vi "FormCalibra6.vi"() -> ()   [LabVIEW 2014]
uses:
  testMachine.ctl
  mainMachine.ctl
  <vilib>/Analysis/baseanly.llb/Mean (DBL).vi
  <vilib>/express/express shared/transition.llb/Dynamic To Waveform Array.vi
  <vilib>/express/express signal manip/GetorSetDDTAttributes/Set DDT Attributes/SetT0.vi
  <vilib>/express/express shared/transition.llb/Waveform Array To Dynamic.vi
  <vilib>/measure/mamon.llb/Trigger Detection for 1 Channel.vi
  <vilib>/express/express signal manip/GetorSetDDTAttributes/Set DDT Attributes/Set DDT Properties.xnode
  <vilib>/Analysis/NI_AALBase.lvlib
  <resource>/objmgr/daqmx.rc
  <vilib>/measure/NI_MAPro.lvlib
panel:
  in  "Lower level":dbl
  in  "hysteresis":dbl format="%.2p"
  in  "level":dbl format="%.2p"
  out "rpm":bool
  out "deviceName":tag
  out "editTotalWaitLimit":u8
  out "editCountWaitLimit":u8
  out "ledWaitState":bool caption="Wait State"
  out "sliderWaitUpperTime":u8(slide) max=50 scale=0.0..100.0
  out "slideWaitLowerTime":u8(slide) max=30 scale=0.0..100.0
  out "slideWaitTime":u8(slide) scale=0.0..100.0
  out "labelTestTime":string caption="Tempo total de ensaio"
  in  "buttonAcquisition":bool
  in  "editSetWaitTime":u8 caption="Tempo entre ciclos (s)" step=1 format="%0d"
  in  "stop":bool
  out "error out":errorcluster
  out "ledAcquireState":bool caption="Acquire State"
  out "editTotalLowerLimit":u8
  out "editCountLowerLimit":u8
  out "editTotalUpperLimit":u8
  out "editCountUpperLimit":u8
  out "ledEnsaio 3":bool
  out "ledBrakeState":bool caption="Brake State"
  out "ledExitState":bool caption="Exit State"
  out "ledMotorState":bool caption="Motor State"
  out "ledInit2State":bool caption="Init State"
  out "ledBlockState":bool caption="Block State"
  out "ledRunningState":bool caption="Running State"
  out "ledReadyState":bool caption="Ready State"
  out "ledInitState":bool caption="Init State"
  out "mainMachine":T1
  out "testMachine":T2=enum."finish"
  in  "editSetPathToFile":path
  in  "buttonStop":bool
  in  "buttonStart":bool
  out "graphForce":dynamicdata(graph)
  in  "editOffsetForce":dbl caption="Tara" min=0.0 max=100.0 step=0.1
  in  "editSetForce":dbl caption="Fator de conversão"
  out "editForce":dbl caption="Força (Kgf)" format="%#_4f"
  out "graphSpeed":dynamicdata(graph)
  in  "editSetSpeed":dbl caption="Fator de conversão"
  out "editSpeed":dbl caption="Velocidade (km/h)" format="%#_4f"
  out "editEngineSpeed":dbl caption="Rotação (RPM)" format="%#_4f"
  in  "buttonMotor":bool
  in  "buttonBrake":bool
  in  "editSetWaitLowerTime":u8 caption="Tempo de espera (s)"
  in  "editSetWaitUpperTime":u8=3 caption="Tempo de espera (s)"
  in  "editSetNumberOfCycles":u16 caption="Número de ciclos" max=999 step=1 format="%0d"
  in  "editSetLowerLimit":u32 caption="Limite inferior (km/h)"
  in  "editSetUpperLimit":u32 caption="Limite superior (km/h)"
  out "editTempB":dbl caption="Temperatura B (ºC)"
  out "editTempA":dbl caption="Temperatura A (ºC)"
  in  "editSetTempRef":dbl caption="Offset referência" step=0.01 format="%#_2f"
  out "editTempRef":dbl caption="Referência (ºC)"
  out "ledMotor":bool
  out "ledBrake":bool
  out "ledEnsaio":bool
  out "labelTotalCycle":string
  out "labelCurrentCycle":string
  out "labelSystemTitle":string
  in  "editCurrCycleCtr":u32
  in  "velocidade 2":u32
  out "velocidade":u32
  # "Bancada de Frenagem - Ensaio"
  # "Ensaio"
  # "Temperatura"
  # "Rotação"
  # "Célula de Carga"
  # "Configurações do ensaio"
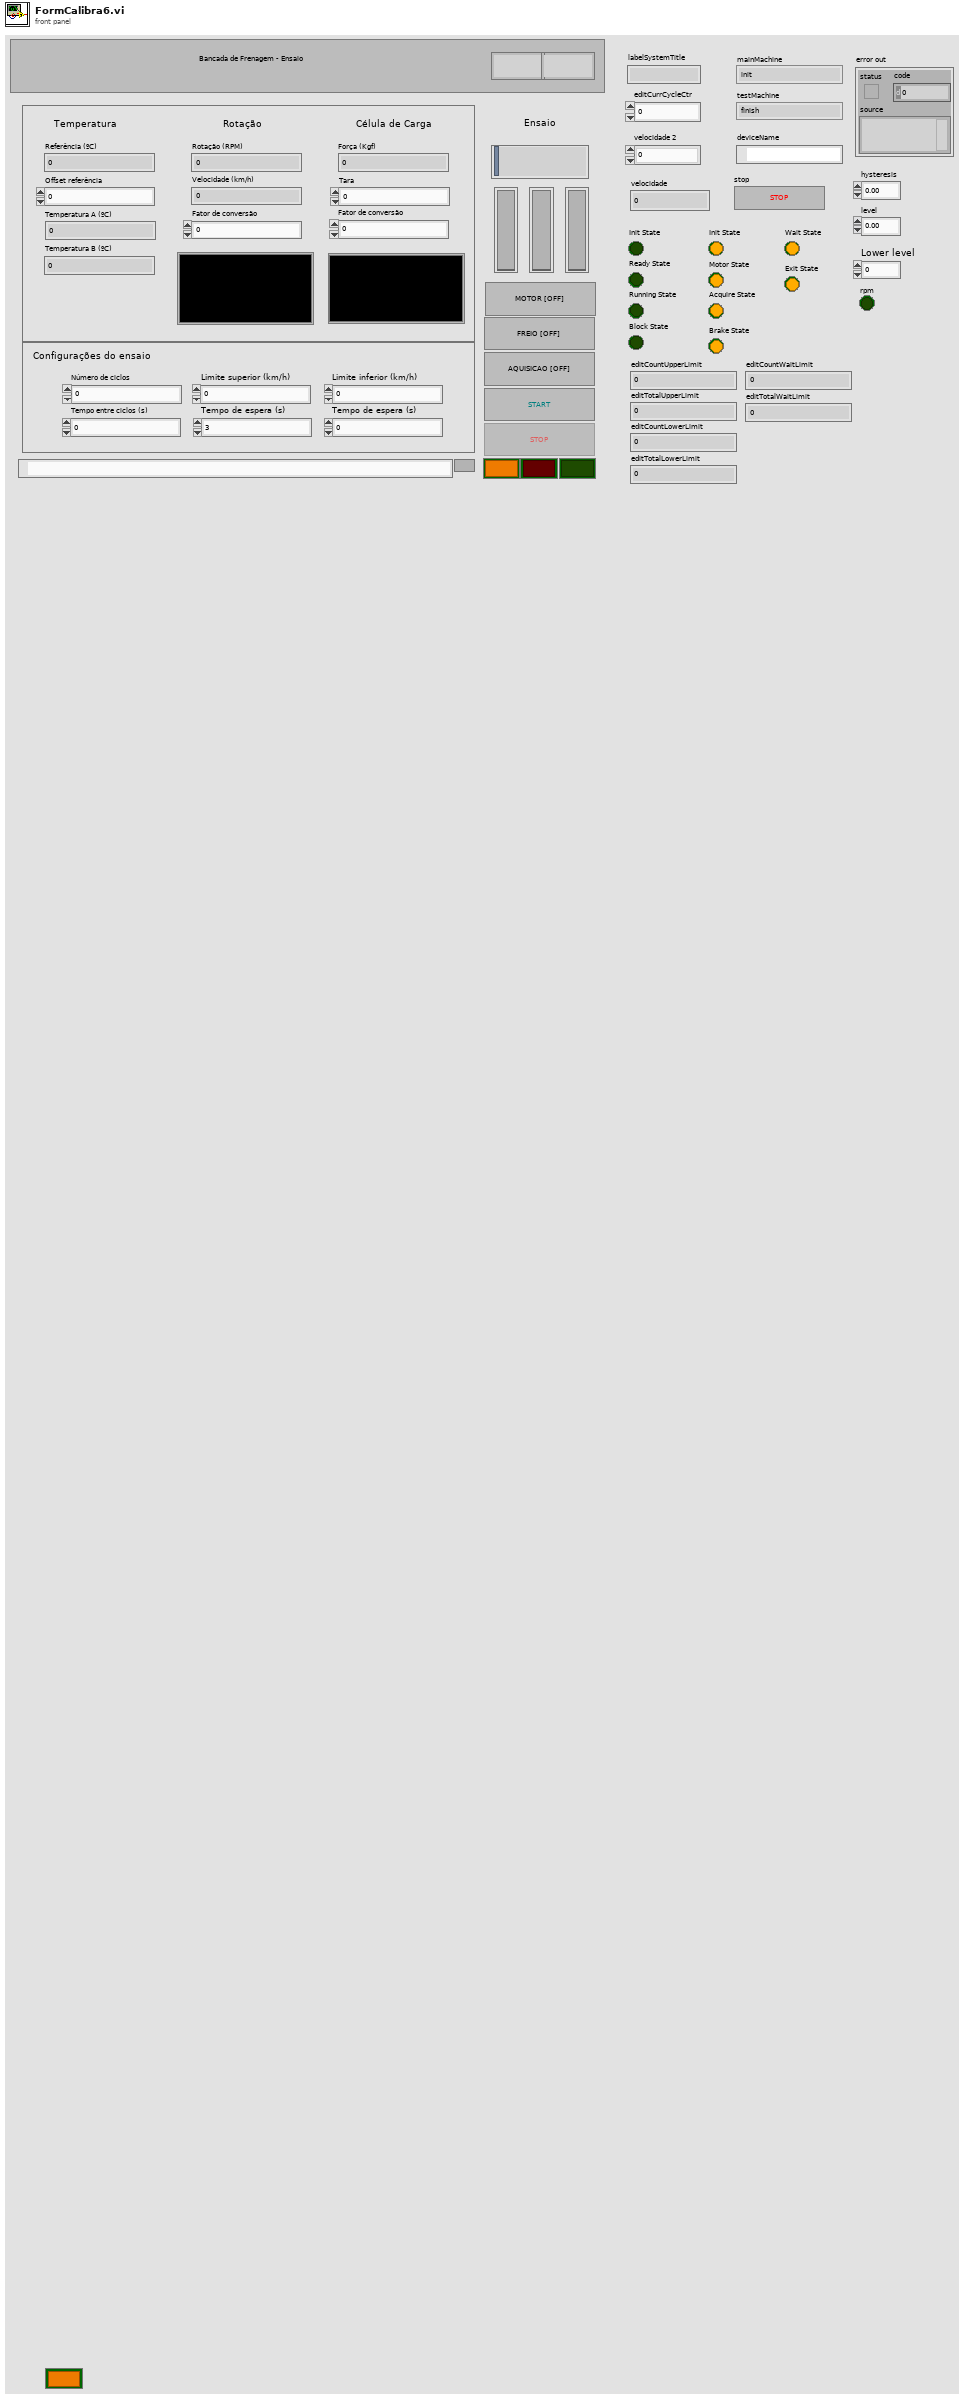
[diagram p1: front panel]
types:
  T1 = typedef "mainMachine.ctl" = enum16{"init", "ready", "running", "blocked", "finish"}
  T2 = typedef "testMachine.ctl" = enum16{"init", "motor", "motor acquire", "brake", "brake acquire", "wait ", "finish", "exit"}
  T3 = enum8{"Enabled", "Disabled", "Disabled and Grayed Out"}
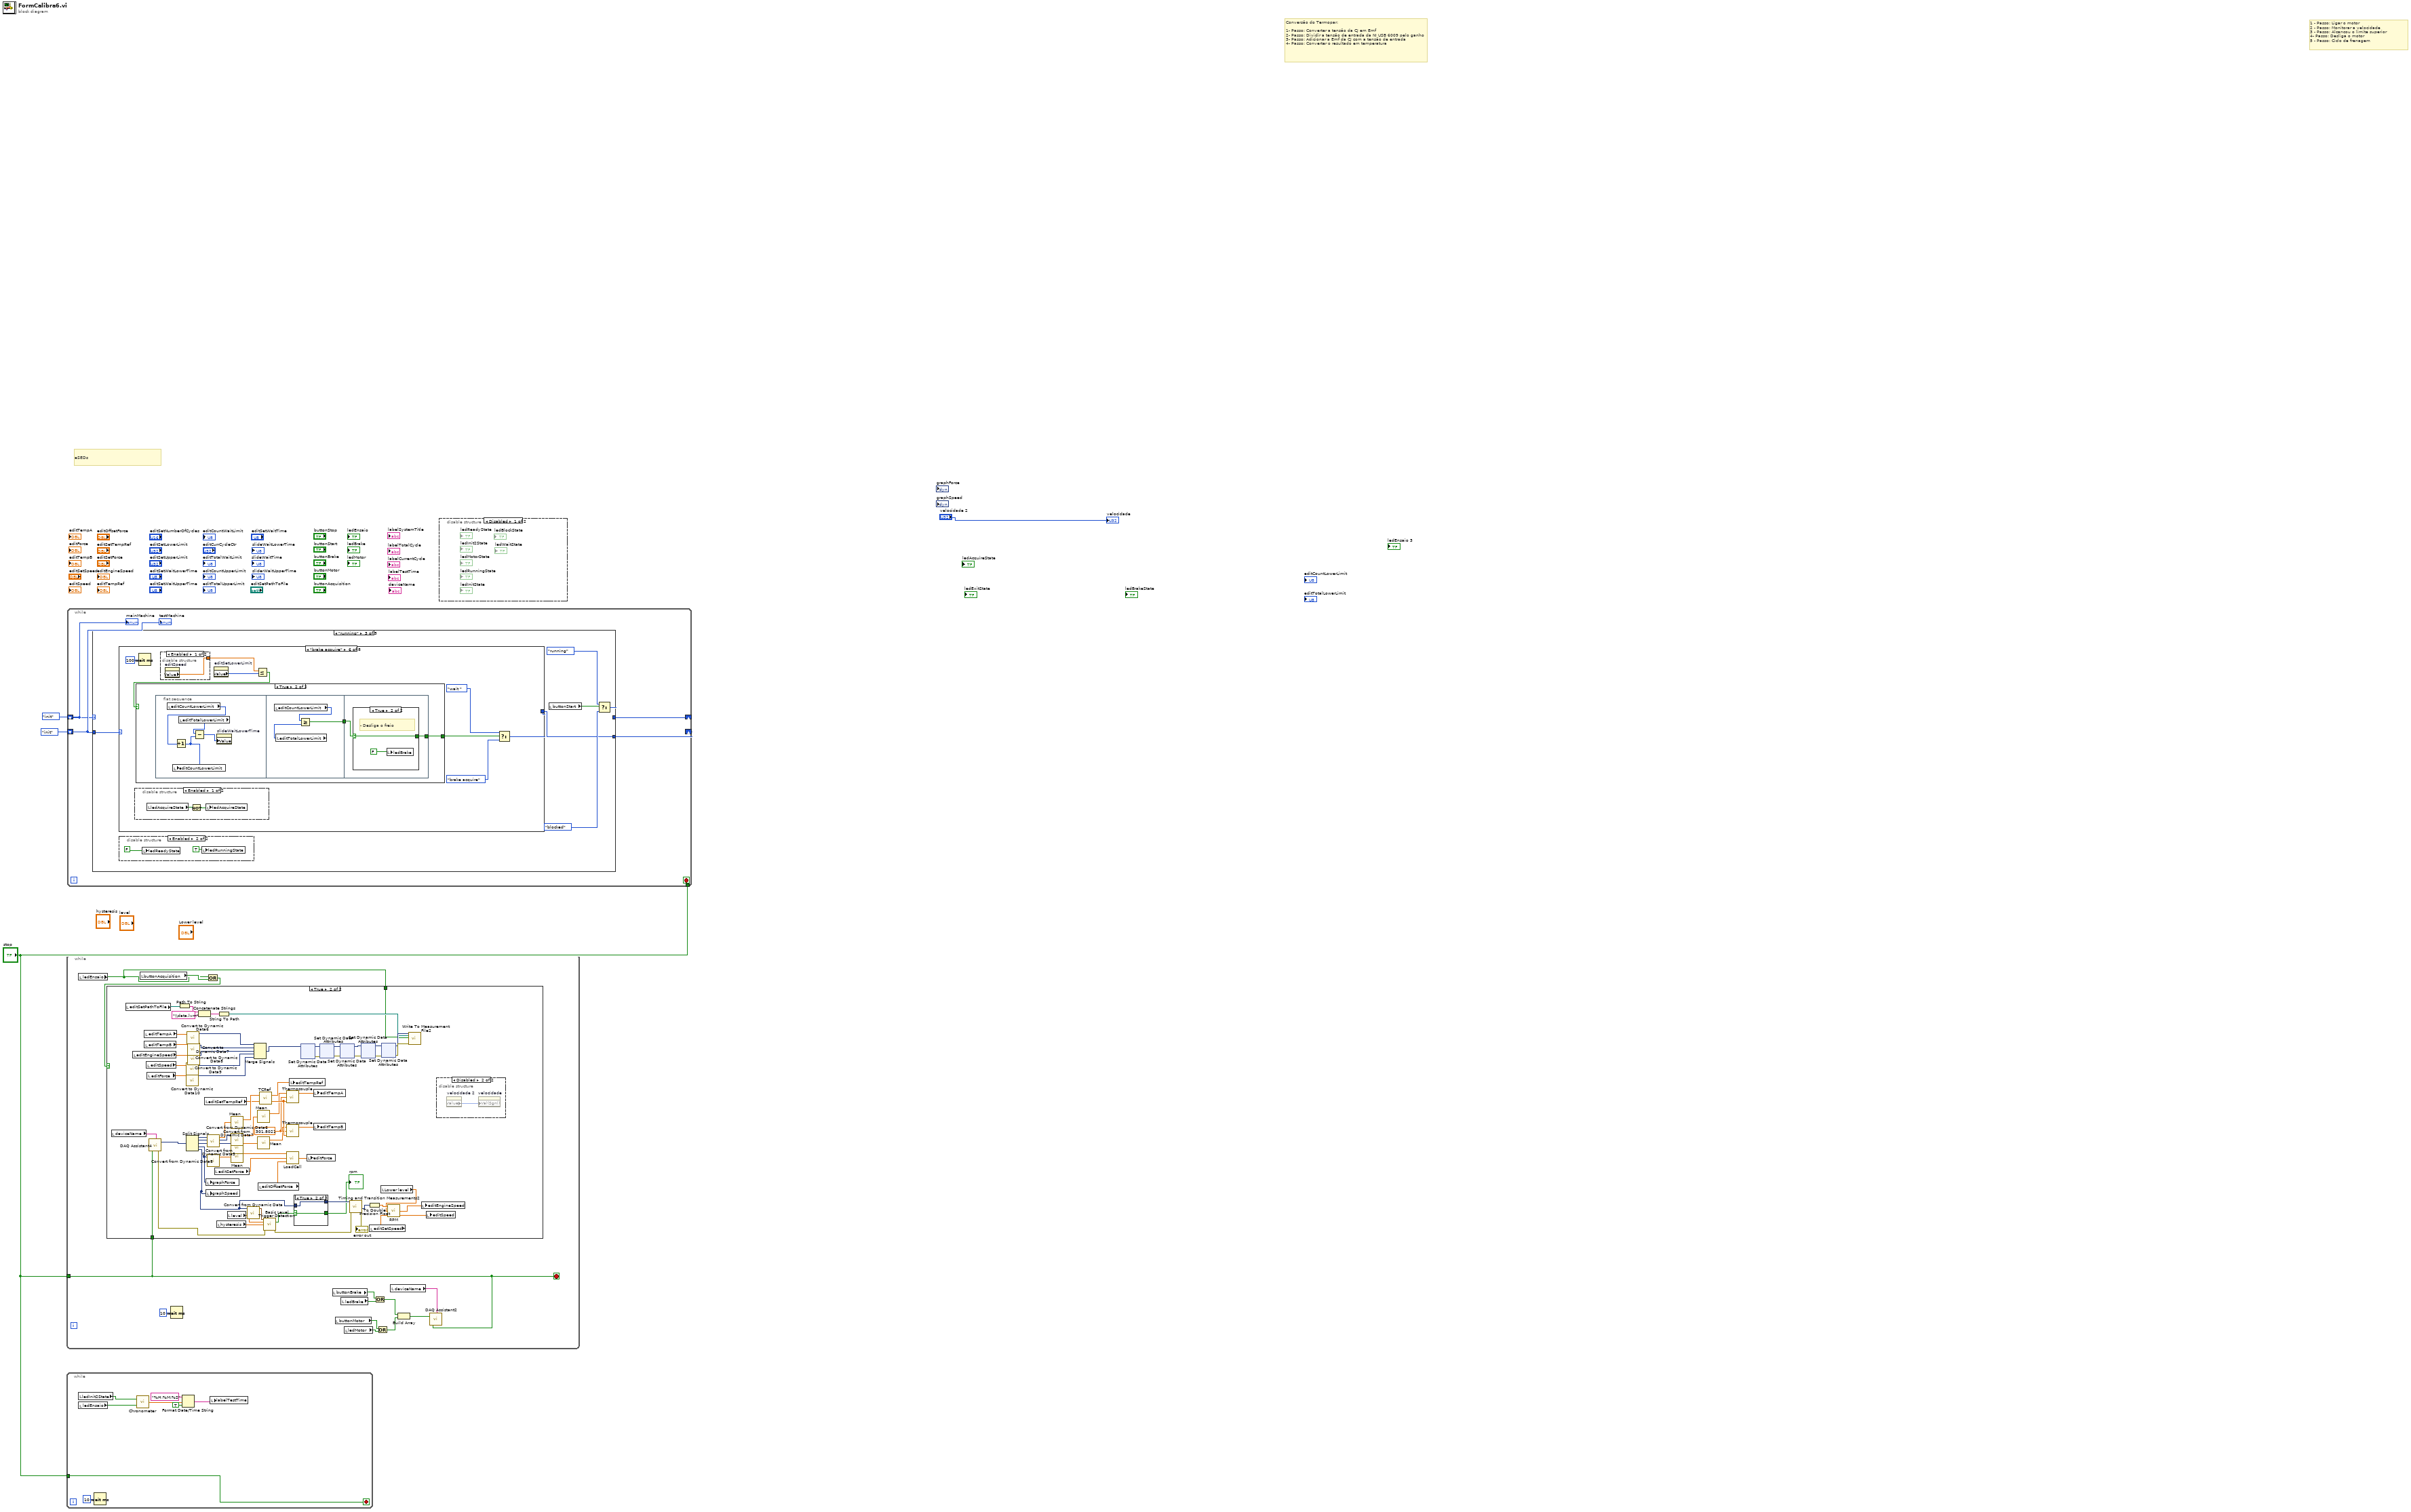
[diagram p0: block diagram]
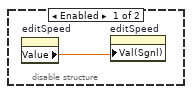
[diagram p5: hidden frame]
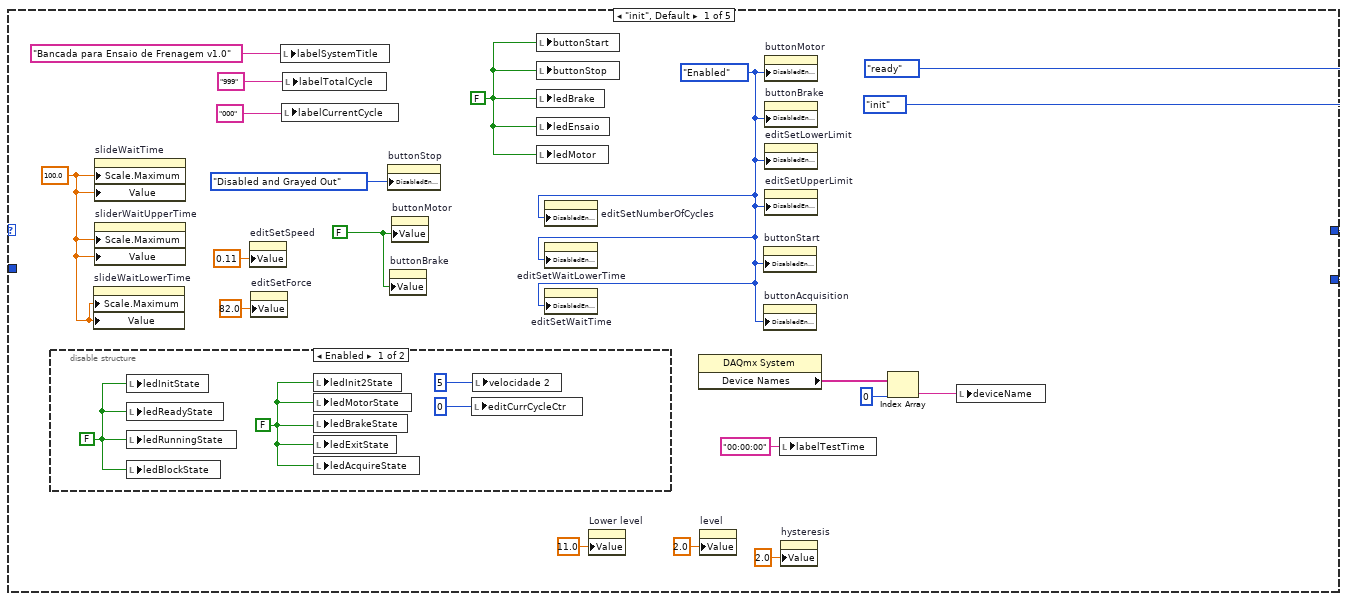
[diagram p6: hidden frame]
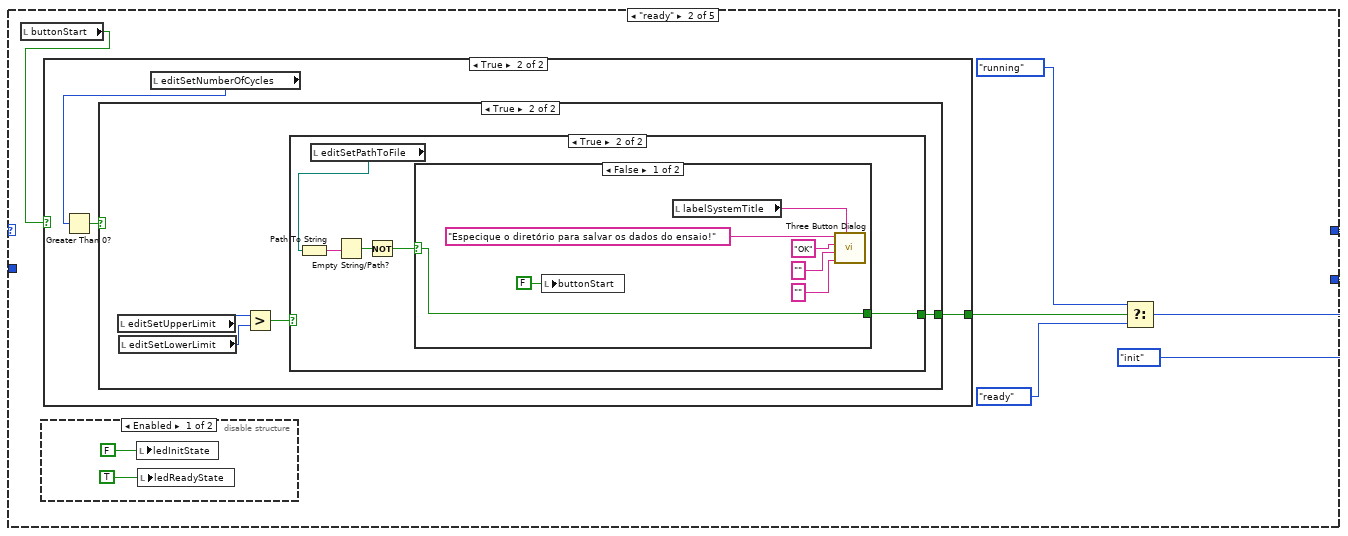
[diagram p8: hidden frame]
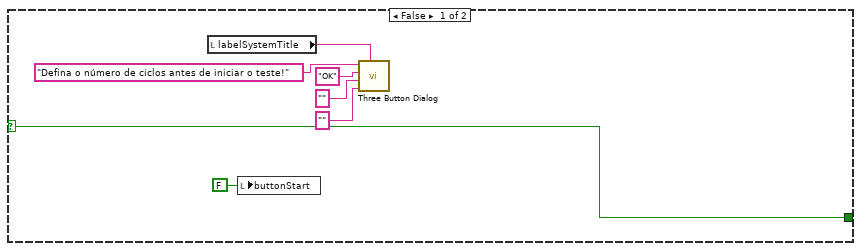
[diagram p11: hidden frame]
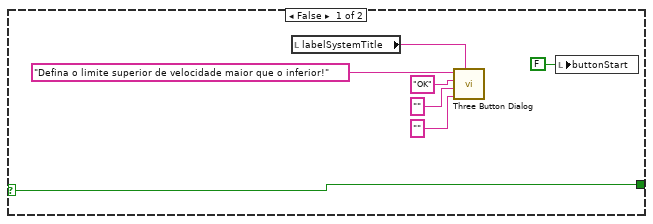
[diagram p12: hidden frame]
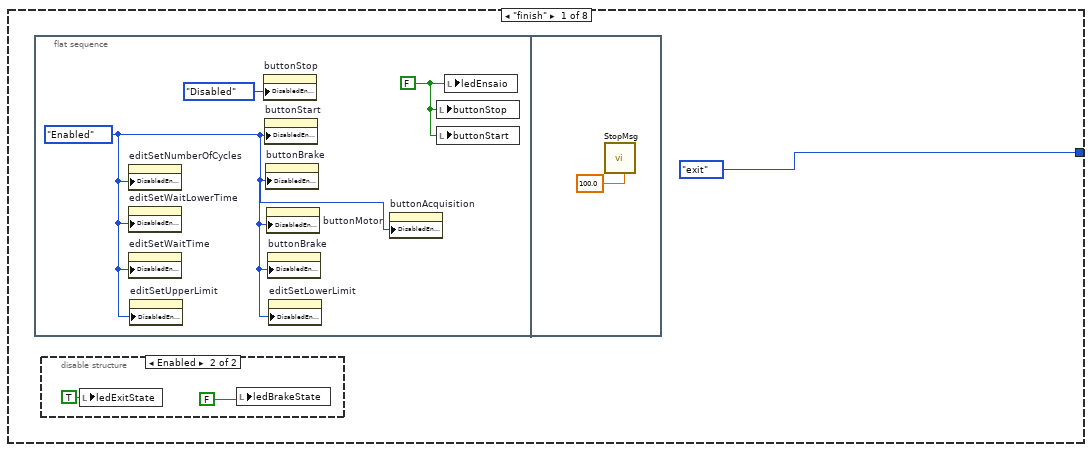
[diagram p15: hidden frame]
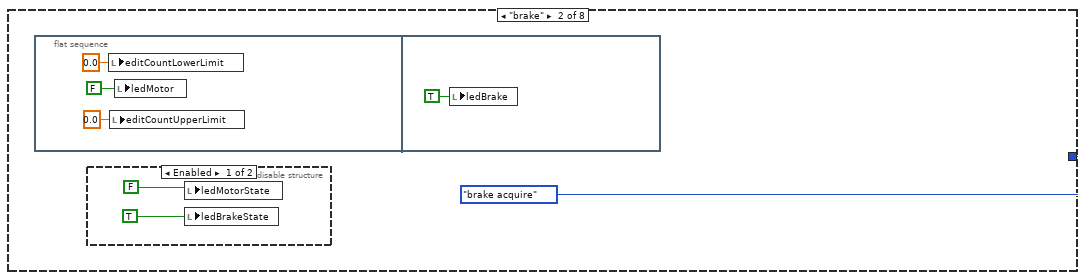
[diagram p17: hidden frame]
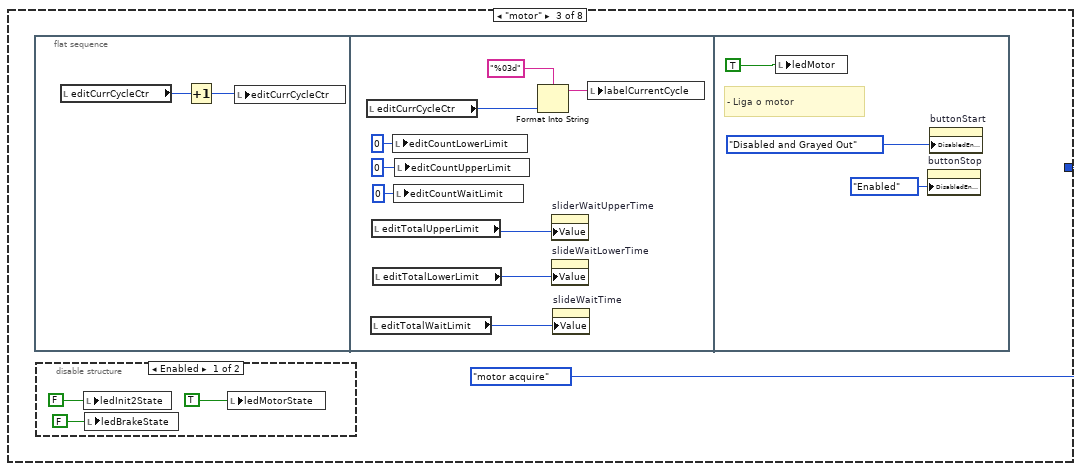
[diagram p19: hidden frame]
diagram:
  # "eSEDs"
  # "1 - Passo: Ligar o motor\n2 - Passo: Monitorar a velocidade\n3 - Passo: Alcancou o limite superior\n4- Passo: Desliga o motor\n5 - Passo: Ciclo de frenagem"
  # "Conversão do Termopar:\n\n1- Passo: Converter a tensão da CJ em Emf\n2- Passo: Dividir a tensão de entrada da NI USB 6009 pelo ganho\n3- Passo: Adicionar a Emf da CJ com a tensão de entrada\n4- Passo: Converter o resultado em temperatura"
  n1 = while {
    tunnel: "stop" -> [w12]
    stop <- w12 stop-if-true
    n2 = local read "ledInit2State"() -> (w6:bool)
    n3 = local read "ledEnsaio"() -> (w5:bool)
    n4 = Wait (ms)(milliseconds to wait=u32 10) -> ()  [unwired: 1 out]
    n5 = call "Chronometer.vi"("start"=w5, "reset"=w6) -> ("Time"=w10:dbl)
    n6 = Format Date/Time String(time format string (%c)="%H:%M:%S", seconds (now)=w10, UTC format=TRUE) -> (date/time string=w7:string)
    n7 = local write "labelTestTime"(w7) -> ()
  }
  n8 = while {
    tunnel: "stop" -> [w18]
    stop <- w18 stop-if-true
    n9 = local read "ledEnsaio"() -> (w15:bool)
    n10 = local read "buttonAcquisition"() -> (w17:bool)
    n11 = Wait (ms)(milliseconds to wait=u32 10) -> ()  [unwired: 1 out]
    n12 = Or(x=w15, y=w17) -> (x .or. y?=w16:bool)
    n13 = case shown="True" w16 {
      tunnel: w18 -> [_ w40]
      tunnel: w15 -> [_ w39]
      frame False {
      }
      frame True {
        w53 = 301.8021 ("factor")
        n14 = local read "deviceName"() -> (w38:tag)
        n15 = local read "editSetPathToFile"() -> (w68:path)
        n16 = local read "editEngineSpeed"() -> (w83:dbl)
        n17 = local read "editTempA"() -> (w80:dbl)
        n18 = local read "editTempB"() -> (w82:dbl)
        n19 = local read "editSpeed"() -> (w84:dbl)
        n20 = local read "editForce"() -> (w85:dbl)
        n21 = call "DAQ Assistant4"("stop (F)"=w40, "device name"=w38) -> ("data"=w42:dynamicdata, "error out"=w37:errorcluster)  [unwired: 14 in, 2 out]
        n22 = Path To String(path=w68) -> (string=w67:string)
        n23 = call "Convert to Dynamic Data9"("Double"=w84) -> ("Dynamic Data Type"=w88:dynamicdata)  [unwired: 3 in]
        n24 = call "Convert to Dynamic Data10"("Double"=w85) -> ("Dynamic Data Type"=w89:dynamicdata)  [unwired: 3 in]
        n25 = Split Signals(w42) -> (w45:dynamicdata, w49:dynamicdata, w47:dynamicdata, w58:dynamicdata, w34:dynamicdata)  [unwired: 5 in]
        n26 = call "Convert to Dynamic Data6"("Double"=w80) -> ("Dynamic Data Type"=w81:dynamicdata)  [unwired: 3 in]
        n27 = call "Convert to Dynamic Data7"("Double"=w82) -> ("Dynamic Data Type"=w86:dynamicdata)  [unwired: 3 in]
        n28 = call "Convert to Dynamic Data8"("Double"=w83) -> ("Dynamic Data Type"=w87:dynamicdata)  [unwired: 3 in]
        n29 = Concatenate Strings(w67, "\\data.lvm" ("string")) -> (w70:string)
        n30 = local read "editSetTempRef"() -> (w44:dbl)
        n31 = local write "graphForce"(w58) -> ()
        n32 = local write "graphSpeed"(w34) -> ()
        n33 = call "Convert from Dynamic Data5"("Dynamic Data Type"=w45) -> ("Array"=w65:dbl[])  [unwired: 3 in]
        n34 = call "Convert from Dynamic Data8"("Dynamic Data Type"=w58) -> ("Array"=w50:dbl[])  [unwired: 3 in]
        n35 = local read "editSetForce"() -> (w63:dbl)
        n36 = local read "hysteresis"() -> (w28:dbl)
        n37 = String To Path(string=w70) -> (path=w71:path)
        n38 = local read "level"() -> (w27:dbl)
        n39 = call-poly <vilib>:"Mean.vi"("X"=w65) -> ("mean"=w66:dbl)  [unwired: 1 out]
        n40 = call "Convert from Dynamic Data6"("Dynamic Data Type"=w49) -> ("Array"=w46:dbl[])  [unwired: 3 in]
        n41 = call "Convert from Dynamic Data7"("Dynamic Data Type"=w47) -> ("Array"=w48:dbl[])  [unwired: 3 in]
        n42 = call-poly <vilib>:"Mean.vi"("X"=w50) -> ("mean"=w57:dbl)  [unwired: 1 out]
        n43 = call "Convert from Dynamic Data"("Dynamic Data Type"=w34) -> ("Waveform"=w33:waveform(dbl))  [unwired: 3 in]
        n44 = Merge Signals(w81, w86, w87, w88, w89) -> (w90:dynamicdata)
        n45 = call-poly <vilib>:"Mean.vi"("X"=w46) -> ("mean"=w51:dbl)  [unwired: 1 out]
        n46 = call-poly <vilib>:"Mean.vi"("X"=w48) -> ("mean"=w52:dbl)  [unwired: 1 out]
        n47 = local read "editOffsetForce"() -> (w64:dbl)
        n48 = call "TCRef.vi"("offset"=w44, "data"=w66) -> ("emf(mV)"=w54:dbl, "temp (degC)"=w43:dbl)
        n49 = call-poly <vilib>:"Basic Level Trigger Detection.vi"("signal in"=w33, "level"=w27, "hysteresis"=w28, "error in (no error)"=w37) -> ("trigger detected?"=w32:bool, "error out"=w36:errorcluster)  [unwired: 9 in, 1 out]
        n50 = call "Thermocouple.vi"("cj(mV)"=w54, "factor"=w53, "data"=w51) -> ("temp(degC)"=w55:dbl)  [unwired: 2 out]
        n51 = call "Thermocouple.vi"("cj(mV)"=w54, "factor"=w53, "data"=w52) -> ("temp(degC)"=w56:dbl)  [unwired: 2 out]
        n52 = call "LoadCell.vi"("tara"=w64, "factor"=w63, "data"=w57) -> ("force (Kgf)"=w60:dbl)
        n53 = local write "editTempRef"(w43) -> ()
        n54 = case shown="True" w32 {
          selector: w32 -> [w93 w94]
          tunnel: w34 -> [_ w95]
          tunnel: [_ w95] -> w35
          tunnel: [w93 w94] -> w31
          frame False {
          }
          frame True {
          }
        }
        "rpm" <- w31
        n55 = xnode ("Set Dynamic Data Attributes")("Signals In"=w90) -> ("Signals Out"=w72:dynamicdata, "error out"=w74:errorcluster)  [unwired: 4 in]
        n56 = local write "editForce"(w60) -> ()
        n57 = local write "editTempA"(w55) -> ()
        n58 = local write "editTempB"(w56) -> ()
        n59 = xnode ("Set Dynamic Data Attributes")("Signals In"=w72, "error in"=w74) -> ("Signals Out"=w73:dynamicdata, "error out"=w75:errorcluster)  [unwired: 3 in]
        n60 = xnode ("Set Dynamic Data Attributes")("Signals In"=w73, "error in"=w75) -> ("Signals Out"=w91:dynamicdata, "error out"=w76:errorcluster)  [unwired: 3 in]
        n61 = call "Timing and Transition Measurements2"("error in (no error)"=w36, "Signals"=w35) -> ("error out"=→"error out":errorcluster, "Frequency"=w30:dynamicdata)  [unwired: 8 in]
        n62 = xnode ("Set Dynamic Data Attributes")("Signals In"=w91, "error in"=w76) -> ("Signals Out"=w92:dynamicdata, "error out"=w77:errorcluster)  [unwired: 3 in]
        n63 = To Double Precision Float(number=w30) -> (double precision float=w29:dbl)
        n64 = local read "editSetSpeed"() -> (w59:dbl)
        n65 = local read "Lower level"() -> (w26:dbl)
        n66 = xnode ("Set Dynamic Data Attributes")("Signals In"=w92, "error in"=w77) -> ("Signals Out"=w78:dynamicdata, "error out"=w79:errorcluster)  [unwired: 3 in]
        n67 = call "RPM.vi"("factor"=w59, "Lower level"=w26, "data"=w29) -> ("km/h"=w62:dbl, "RPM"=w61:dbl)  [unwired: 1 out]
        n68 = call "Write To Measurement File2"("Signals"=w78, "Enable"=w39, "error in (no error)"=w79, "Filename"=w71) -> ()  [unwired: 13 in, 3 out]
        n69 = local write "editEngineSpeed"(w61) -> ()
        n70 = local write "editSpeed"(w62) -> ()
        n71 = disable-structure shown="Disabled" {
          frame Enabled {
            n72 = property on="editSpeed" class="DigNum (strict)"() -> ("Value"=w96:dbl)  [unwired: 2 in, 2 out]
            n73 = property on="editSpeed" class="DigNum (strict)"("Val(Sgnl)"=w96) -> ()  [unwired: 2 in, 2 out]
          }
          frame Disabled {
            n74 = property on="velocidade 2" class="DigNum (strict)"() -> ("Value"=w97:u32)  [unwired: 2 in, 2 out]
            n75 = property on="velocidade" class="DigNum (strict)"("Val(Sgnl)"=w97) -> ()  [unwired: 2 in, 2 out]
          }
        }
      }
    }
    n76 = local read "buttonBrake"() -> (w22:bool)
    n77 = local read "buttonMotor"() -> (w20:bool)
    n78 = local read "ledBrake"() -> (w24:bool)
    n79 = local read "ledMotor"() -> (w21:bool)
    n80 = Or(x=w22, y=w24) -> (x .or. y?=w23:bool)
    n81 = Or(x=w20, y=w21) -> (x .or. y?=w19:bool)
    n82 = local read "deviceName"() -> (w13:tag)
    n83 = Build Array(w23, w19) -> (w25:bool[])
    n84 = call "DAQ Assistant2"("data"=w25, "stop (T)"=w18, "device name"=w13) -> ()  [unwired: 15 in, 2 out]
  }
  n85 = while {
    shift-right: [w192] -> _
    shift-left: mainMachine."init" ("mainMachine") -> [w189]
    shift-right: [w191] -> _
    shift-left: testMachine."init" ("testMachine") -> [w190]
    tunnel: "stop" -> [w188]
    stop <- w188 stop-if-true
    n86 = case shown="\"running\"" w189 {
      tunnel: [mainMachine."ready" ("mainMachine") w216 w261 w401 mainMachine."finish" ("mainMachine")] -> w192
      tunnel: [testMachine."init" ("testMachine") testMachine."init" ("testMachine") w260 testMachine."init" ("testMachine") testMachine."init" ("testMachine")] -> w191
      tunnel: w190 -> [_ _ w259 _ _]
      frame "init", Default {
        w202 = 100.0 ("Scale.Range:Maximum")
        w203 = T3."Enabled" ("Disabled")
        w204 = FALSE ("buttonMotor")
        w210 = FALSE ("motor")
        n87 = disable-structure shown="Enabled" {
          frame Enabled {
            w212 = FALSE
            w213 = FALSE
            n88 = local write "ledInitState"(w213) -> ()
            n89 = local write "ledReadyState"(w213) -> ()
            n90 = local write "ledRunningState"(w213) -> ()
            n91 = local write "ledBlockState"(w213) -> ()
            n92 = local write "ledInit2State"(w212) -> ()
            n93 = local write "ledMotorState"(w212) -> ()
            n94 = local write "ledBrakeState"(w212) -> ()
            n95 = local write "ledExitState"(w212) -> ()
            n96 = local write "ledAcquireState"(w212) -> ()
            n97 = local write "editCurrCycleCtr"(u32 0 ("currentCycleCtr")) -> ()
            n98 = local write "velocidade 2"(u32 5 ("velocidade 2")) -> ()
          }
          frame Disabled {
          }
        }
        n99 = property on="slideWaitLowerTime" class="Slide (strict)"("Scale.Maximum"=w202, "Value"=w202) -> ()  [unwired: 2 in, 2 out]
        n100 = property on="slideWaitTime" class="Slide (strict)"("Scale.Maximum"=w202, "Value"=w202) -> ()  [unwired: 2 in, 2 out]
        n101 = property on="sliderWaitUpperTime" class="Slide (strict)"("Scale.Maximum"=w202, "Value"=w202) -> ()  [unwired: 2 in, 2 out]
        n102 = property on="editSetSpeed" class="DigNum (strict)"("Value"=0.11 ("editSetSpeed")) -> ()  [unwired: 2 in, 2 out]
        n103 = property on="editSetForce" class="DigNum (strict)"("Value"=82.0 ("editSetForce")) -> ()  [unwired: 2 in, 2 out]
        n104 = local write "labelSystemTitle"("Bancada para Ensaio de Frenagem v1.0" ("systemTitle")) -> ()
        n105 = local write "labelCurrentCycle"("000" ("currentCycle")) -> ()
        n106 = local write "labelTotalCycle"("999" ("totalCycle")) -> ()
        n107 = property on="buttonStop" class="Bool (strict)"("DisabledEnum"=T3."Disabled and Grayed Out" ("Disabled")) -> ()  [unwired: 2 in, 2 out]
        n108 = property on="buttonBrake" class="Bool (strict)"("Value"=w204) -> ()  [unwired: 2 in, 2 out]
        n109 = property on="buttonMotor" class="Bool (strict)"("Value"=w204) -> ()  [unwired: 2 in, 2 out]
        n110 = local write "buttonStart"(w210) -> ()
        n111 = local write "buttonStop"(w210) -> ()
        n112 = local write "ledBrake"(w210) -> ()
        n113 = local write "ledEnsaio"(w210) -> ()
        n114 = local write "ledMotor"(w210) -> ()
        n115 = property on="editSetNumberOfCycles" class="DigNum (strict)"("DisabledEnum"=w203) -> ()  [unwired: 2 in, 2 out]
        n116 = property on="editSetWaitLowerTime" class="DigNum (strict)"("DisabledEnum"=w203) -> ()  [unwired: 2 in, 2 out]
        n117 = property on="editSetWaitTime" class="DigNum (strict)"("DisabledEnum"=w203) -> ()  [unwired: 2 in, 2 out]
        n118 = property on="Lower level" class="DigNum (strict)"("Value"=11.0 ("Lower level")) -> ()  [unwired: 2 in, 2 out]
        n119 = property class="DAQmx System"() -> ("Device Names"=w201:tag[])  [unwired: 2 in, 2 out]
        n120 = property on="level" class="DigNum (strict)"("Value"=2.0 ("level")) -> ()  [unwired: 2 in, 2 out]
        n121 = property on="buttonStart" class="Bool (strict)"("DisabledEnum"=w203) -> ()  [unwired: 2 in, 2 out]
        n122 = property on="buttonAcquisition" class="Bool (strict)"("DisabledEnum"=w203) -> ()  [unwired: 2 in, 2 out]
        n123 = property on="buttonMotor" class="Bool (strict)"("DisabledEnum"=w203) -> ()  [unwired: 2 in, 2 out]
        n124 = property on="buttonBrake" class="Bool (strict)"("DisabledEnum"=w203) -> ()  [unwired: 2 in, 2 out]
        n125 = property on="editSetLowerLimit" class="DigNum (strict)"("DisabledEnum"=w203) -> ()  [unwired: 2 in, 2 out]
        n126 = property on="editSetUpperLimit" class="DigNum (strict)"("DisabledEnum"=w203) -> ()  [unwired: 2 in, 2 out]
        n127 = local write "labelTestTime"("00:00:00" ("labelTestTime")) -> ()
        n128 = property on="hysteresis" class="DigNum (strict)"("Value"=2.0 ("hysteresis")) -> ()  [unwired: 2 in, 2 out]
        n129 = Index Array(array=w201, index=0) -> (element=w199:tag)
        n130 = local write "deviceName"(w199) -> ()
      }
      frame "ready" {
        n131 = local read "buttonStart"() -> (w219:bool)
        n132 = disable-structure shown="Enabled" {
          frame Enabled {
            n133 = local write "ledInitState"(FALSE ("ledReady")) -> ()
            n134 = local write "ledReadyState"(TRUE ("ledReady")) -> ()
          }
          frame Disabled {
          }
        }
        n135 = case shown="True" w219 {
          selector: w219 -> [w224 _]
          tunnel: [w224 w225] -> w218
          frame False {
          }
          frame True {
            n136 = local read "editSetNumberOfCycles"() -> (w226:u16)
            n137 = Greater Than 0?(x=w226) -> (x > 0?=w227:bool)
            n138 = case shown="True" w227 {
              selector: w227 -> [w234 _]
              tunnel: [w234 w235] -> w225
              frame False {
                n139 = local read "labelSystemTitle"() -> (w229:string)
                n140 = local write "buttonStart"(FALSE ("startButton")) -> ()
                n141 = call <vilib>:"Three Button Dialog.vi"("Window Title (\"\")"=w229, "Right Button Text (\"Cancel\")"="" ("Right Button Text (\"Cancel\")"), "Center Button Text (\"No\")"="" ("Center Button Text (\"No\")"), "Left Button Text (\"Yes\")"="OK" ("Left Button Text (\"Yes\")"), "message"="Defina o número de ciclos antes de iniciar o teste!") -> ()  [unwired: 6 in, 1 out]
              }
              frame True {
                n142 = local read "editSetUpperLimit"() -> (w237:u32)
                n143 = local read "editSetLowerLimit"() -> (w236:u32)
                n144 = Greater?(x=w237, y=w236) -> (0:w238:bool)
                n145 = case shown="True" w238 {
                  selector: w238 -> [w245 _]
                  tunnel: [w245 w248] -> w235
                  frame False {
                    n146 = local read "labelSystemTitle"() -> (w240:string)
                    n147 = call <vilib>:"Three Button Dialog.vi"("Window Title (\"\")"=w240, "Right Button Text (\"Cancel\")"="" ("Right Button Text (\"Cancel\")"), "Center Button Text (\"No\")"="" ("Center Button Text (\"No\")"), "Left Button Text (\"Yes\")"="OK" ("Left Button Text (\"Yes\")"), "message"="Defina o limite superior de velocidade maior que o inferior!") -> ()  [unwired: 6 in, 1 out]
                    n148 = local write "buttonStart"(FALSE ("startButton")) -> ()
                  }
                  frame True {
                    n149 = local read "editSetPathToFile"() -> (w250:path)
                    n150 = Path To String(path=w250) -> (string=w249:string)
                    n151 = Empty String/Path?(string/path=w249) -> (empty?=w247:bool)
                    n152 = Not(x=w247) -> (.not. x?=w246:bool)
                    n153 = case shown="False" w246 {
                      selector: w246 -> [w257 w258]
                      tunnel: [w257 w258] -> w248
                      frame False {
                        n154 = local write "buttonStart"(FALSE ("startButton")) -> ()
                        n155 = local read "labelSystemTitle"() -> (w252:string)
                        n156 = call <vilib>:"Three Button Dialog.vi"("Window Title (\"\")"=w252, "Right Button Text (\"Cancel\")"="" ("Right Button Text (\"Cancel\")"), "Center Button Text (\"No\")"="" ("Center Button Text (\"No\")"), "Left Button Text (\"Yes\")"="OK" ("Left Button Text (\"Yes\")"), "message"="Especique o diretório para salvar os dados do ensaio!") -> ()  [unwired: 6 in, 1 out]
                      }
                      frame True {
                      }
                    }
                  }
                }
              }
            }
          }
        }
        n157 = Select(t=mainMachine."running" ("mainMachine"), s=w218, f=mainMachine."ready" ("mainMachine")) -> (s? t:f=w216:T1)
      }
      frame "running" {
        n158 = case shown="\"brake acquire\"" w259 {
          tunnel: [testMachine."exit" ("testMachine") testMachine."brake acquire" ("testMachine") testMachine."motor acquire" ("testMachine") testMachine."motor" ("testMachine") w331 w351 testMachine."exit" ("testMachine") w384] -> w260
          frame "finish" {
            n159 = flat-sequence {
              frame #0 {
                w271 = FALSE ("ledReady")
                w270 = T3."Enabled" ("Disabled")
                n160 = property on="editSetNumberOfCycles" class="DigNum (strict)"("DisabledEnum"=w270) -> ()  [unwired: 2 in, 2 out]
                n161 = property on="editSetWaitLowerTime" class="DigNum (strict)"("DisabledEnum"=w270) -> ()  [unwired: 2 in, 2 out]
                n162 = property on="editSetWaitTime" class="DigNum (strict)"("DisabledEnum"=w270) -> ()  [unwired: 2 in, 2 out]
                n163 = property on="editSetUpperLimit" class="DigNum (strict)"("DisabledEnum"=w270) -> ()  [unwired: 2 in, 2 out]
                n164 = property on="buttonStop" class="Bool (strict)"("DisabledEnum"=T3."Disabled" ("Disabled")) -> ()  [unwired: 2 in, 2 out]
                n165 = property on="buttonStart" class="Bool (strict)"("DisabledEnum"=w270) -> ()  [unwired: 2 in, 2 out]
                n166 = property on="buttonBrake" class="Bool (strict)"("DisabledEnum"=w270) -> ()  [unwired: 2 in, 2 out]
                n167 = property on="buttonMotor" class="Bool (strict)"("DisabledEnum"=w270) -> ()  [unwired: 2 in, 2 out]
                n168 = property on="buttonBrake" class="Bool (strict)"("DisabledEnum"=w270) -> ()  [unwired: 2 in, 2 out]
                n169 = property on="editSetLowerLimit" class="DigNum (strict)"("DisabledEnum"=w270) -> ()  [unwired: 2 in, 2 out]
                n170 = property on="buttonAcquisition" class="Bool (strict)"("DisabledEnum"=w270) -> ()  [unwired: 2 in, 2 out]
                n171 = local write "buttonStop"(w271) -> ()
                n172 = local write "buttonStart"(w271) -> ()
                n173 = local write "ledEnsaio"(w271) -> ()
              }
              frame #1 {
                n174 = call "StopMsg.vi"("Max Value (100)"=100.0) -> ()  [unwired: 8 in, 2 out]
              }
            }
            n175 = disable-structure shown="Enabled" {
              frame Disabled {
              }
              frame Enabled {
                n176 = local write "ledExitState"(TRUE ("ledReady")) -> ()
                n177 = local write "ledBrakeState"(FALSE ("ledReady")) -> ()
              }
            }
          }
          frame "brake" {
            n178 = flat-sequence {
              frame #0 {
                n179 = local write "editCountLowerLimit"(0.0 ("editCountUpperLimit")) -> ()
                n180 = local write "editCountUpperLimit"(0.0 ("editCountUpperLimit")) -> ()
                n181 = local write "ledMotor"(FALSE ("motor")) -> ()
              }
              frame #1 {
                n182 = local write "ledBrake"(TRUE ("freio")) -> ()
              }
            }
            n183 = disable-structure shown="Enabled" {
              frame Enabled {
                n184 = local write "ledMotorState"(FALSE ("ledReady")) -> ()
                n185 = local write "ledBrakeState"(TRUE ("ledReady")) -> ()
              }
              frame Disabled {
              }
            }
          }
          frame "motor" {
            n186 = flat-sequence {
              frame #0 {
                n187 = local read "editCurrCycleCtr"() -> (w286:u32)
                n188 = Increment(x=w286) -> (x+1=w285:u32)
                n189 = local write "editCurrCycleCtr"(w285) -> ()
              }
              frame #1 {
                n190 = local read "editCurrCycleCtr"() -> (w293:u32)
                n191 = local read "editTotalWaitLimit"() -> (w287:u8)
                n192 = local read "editTotalUpperLimit"() -> (w289:u8)
                n193 = local read "editTotalLowerLimit"() -> (w288:u8)
                n194 = local write "editCountLowerLimit"(u8 0 ("editCountLowerLimit")) -> ()
                n195 = local write "editCountWaitLimit"(u8 0 ("editCountWaitLimit")) -> ()
                n196 = local write "editCountUpperLimit"(u8 0 ("editCountUpperLimit")) -> ()
                n197 = Format Into String(format string="%03d", w293) -> (resulting string=w294:string)  [unwired: 2 in, 1 out]
                n198 = property on="sliderWaitUpperTime" class="Slide (strict)"("Value"=w289) -> ()  [unwired: 2 in, 2 out]
                n199 = property on="slideWaitLowerTime" class="Slide (strict)"("Value"=w288) -> ()  [unwired: 2 in, 2 out]
                n200 = property on="slideWaitTime" class="Slide (strict)"("Value"=w287) -> ()  [unwired: 2 in, 2 out]
                n201 = local write "labelCurrentCycle"(w294) -> ()
              }
              frame #2 {
                # "- Liga o motor"
                n202 = local write "ledMotor"(TRUE ("motor")) -> ()
                n203 = property on="buttonStop" class="Bool (strict)"("DisabledEnum"=T3."Enabled" ("Disabled")) -> ()  [unwired: 2 in, 2 out]
                n204 = property on="buttonStart" class="Bool (strict)"("DisabledEnum"=T3."Disabled and Grayed Out" ("Disabled")) -> ()  [unwired: 2 in, 2 out]
              }
            }
            n205 = disable-structure shown="Enabled" {
              frame Enabled {
                n206 = local write "ledInit2State"(FALSE ("ledReady")) -> ()
                n207 = local write "ledBrakeState"(FALSE ("ledReady")) -> ()
                n208 = local write "ledMotorState"(TRUE ("ledReady")) -> ()
              }
              frame Disabled {
              }
            }
          }
          frame "init", Default {
            n209 = stacked-sequence {
              frame #0 {
                w306 = FALSE ("ensaio")
                n210 = property on="buttonBrake" class="Bool (strict)"("Value"=w306) -> ()  [unwired: 2 in, 2 out]
                n211 = local write "ledMotor"(w306) -> ()
                n212 = local write "ledBrake"(w306) -> ()
                n213 = property on="buttonMotor" class="Bool (strict)"("Value"=w306) -> ()  [unwired: 2 in, 2 out]
                n214 = local read "editSetNumberOfCycles"() -> (w313:u16)
                n215 = local read "editSetWaitLowerTime"() -> (w307:u8)
                n216 = local read "editSetWaitUpperTime"() -> (w310:u8)
                n217 = local read "editSetWaitTime"() -> (w301:u8)
                n218 = Multiply(x=w301, y=u32 10) -> (x*y=w302:u32)
                n219 = Multiply(x=w307, y=u32 10) -> (x*y=w305:u32)
                n220 = Format Into String(format string="%03d", w313) -> (resulting string=w314:string)  [unwired: 2 in, 1 out]
                n221 = Multiply(x=w310, y=u32 10) -> (x*y=w304:u32)
                n222 = local write "editTotalLowerLimit"(w305) -> ()
                n223 = local write "editTotalUpperLimit"(w304) -> ()
                n224 = local write "editTotalWaitLimit"(w302) -> ()
                n225 = local write "labelTotalCycle"(w314) -> ()
                n226 = local write "editCurrCycleCtr"(u32 0 ("currentCycleCtr")) -> ()
                n227 = local write "labelCurrentCycle"("000" ("currentCycle")) -> ()
              }
              frame #1 {
                w322 = T3."Disabled" ("Disabled")
                n228 = property on="editSetNumberOfCycles" class="DigNum (strict)"("DisabledEnum"=w322) -> ()  [unwired: 2 in, 2 out]
                n229 = property on="editSetWaitLowerTime" class="DigNum (strict)"("DisabledEnum"=w322) -> ()  [unwired: 2 in, 2 out]
                n230 = property on="editSetWaitTime" class="DigNum (strict)"("DisabledEnum"=w322) -> ()  [unwired: 2 in, 2 out]
                n231 = local read "editTotalUpperLimit"() -> (w325:u8)
                n232 = property on="sliderWaitUpperTime" class="Slide (strict)"("Scale.Maximum"=w325, "Scale.Minimum"=0.0 ("Scale.Range:Minimum"), "Scale.Increment"=1.0 ("Scale.Range:Increment"), "Value"=w325) -> ()  [unwired: 2 in, 2 out]
                n233 = property on="buttonAcquisition" class="Bool (strict)"("DisabledEnum"=w322) -> ()  [unwired: 2 in, 2 out]
                n234 = local read "editTotalLowerLimit"() -> (w319:u8)
                n235 = property on="slideWaitLowerTime" class="Slide (strict)"("Scale.Maximum"=w319, "Scale.Minimum"=0.0 ("Scale.Range:Minimum"), "Scale.Increment"=1.0 ("Scale.Range:Increment"), "Value"=w319) -> ()  [unwired: 2 in, 2 out]
                n236 = local read "editTotalWaitLimit"() -> (w316:u8)
                n237 = property on="slideWaitTime" class="Slide (strict)"("Scale.Maximum"=w316, "Scale.Minimum"=0.0 ("Scale.Range:Minimum"), "Scale.Increment"=1.0 ("Scale.Range:Increment"), "Value"=w316) -> ()  [unwired: 2 in, 2 out]
                n238 = call "StarMsg.vi"("Show"=TRUE, "Max Value (100)"=100.0) -> ()  [unwired: 7 in, 2 out]
                n239 = property on="buttonMotor" class="Bool (strict)"("DisabledEnum"=w322) -> ()  [unwired: 2 in, 2 out]
                n240 = property on="buttonBrake" class="Bool (strict)"("DisabledEnum"=w322) -> ()  [unwired: 2 in, 2 out]
                n241 = property on="editSetLowerLimit" class="DigNum (strict)"("DisabledEnum"=w322) -> ()  [unwired: 2 in, 2 out]
                n242 = property on="editSetUpperLimit" class="DigNum (strict)"("DisabledEnum"=w322) -> ()  [unwired: 2 in, 2 out]
              }
              frame #2 {
                n243 = local write "ledEnsaio"(TRUE ("ensaio")) -> ()
              }
            }
            n244 = disable-structure shown="Enabled" {
              frame Enabled {
                n245 = local write "ledInit2State"(TRUE ("ledReady")) -> ()
              }
              frame Disabled {
              }
            }
          }
          frame "motor acquire" {
            n246 = disable-structure shown="Enabled" {
              frame Enabled {
                n247 = local read "ledAcquireState"() -> (w340:bool)
                n248 = Not(x=w340) -> (.not. x?=w339:bool)
                n249 = local write "ledAcquireState"(w339) -> ()
              }
              frame Disabled {
              }
            }
            n250 = Wait (ms)(milliseconds to wait=u32 100) -> ()  [unwired: 1 out]
            n251 = disable-structure shown="Enabled" {
              disable-tunnel: [w337 w338] -> w330
              frame Enabled {
                n252 = property on="editSpeed" class="DigNum (strict)"() -> ("Value"=w337:dbl)  [unwired: 2 in, 2 out]
              }
              frame Disabled {
                n253 = property on="velocidade" class="DigNum (strict)"() -> ("Value"=w338:u32)  [unwired: 2 in, 2 out]
              }
            }
            n254 = property on="editSetUpperLimit" class="DigNum (strict)"() -> ("Value"=w329:u32)  [unwired: 2 in, 2 out]
            n255 = Greater Or Equal?(x=w330, y=w329) -> (x >= y?=w335:bool)
            n256 = case shown="True" w335 {
              selector: w335 -> [w341 _]
              tunnel: [w341 w342] -> w334
              frame False {
              }
              frame True {
                n257 = flat-sequence {
                  tunnel: [w347] -> w342
                  frame #0 {
                    n258 = local read "editCountUpperLimit"() -> (w345:u8)
                    n259 = Increment(x=w345) -> (x+1=w343:u8)
                    n260 = local write "editCountUpperLimit"(w343) -> ()
                    n261 = local read "editTotalUpperLimit"() -> (w344:u8)
                    n262 = Subtract(x=w344, y=w343) -> (x-y=w346:u8)
                    n263 = property on="sliderWaitUpperTime" class="Slide (strict)"("Value"=w346) -> ()  [unwired: 2 in, 2 out]
                  }
                  frame #1 {
                    n264 = local read "editCountUpperLimit"() -> (w349:u8)
                    n265 = local read "editTotalUpperLimit"() -> (w348:u8)
                    n266 = Greater Or Equal?(x=w349, y=w348) -> (x >= y?=w347:bool)
                  }
                }
              }
            }
            n267 = Select(t=testMachine."brake" ("testMachine"), s=w334, f=testMachine."motor acquire" ("testMachine")) -> (s? t:f=w331:T2)
          }
          frame "brake acquire" {
            n268 = disable-structure shown="Enabled" {
              frame Enabled {
                n269 = local read "ledAcquireState"() -> (w359:bool)
                n270 = Not(x=w359) -> (.not. x?=w358:bool)
                n271 = local write "ledAcquireState"(w358) -> ()
              }
              frame Disabled {
              }
            }
            n272 = Wait (ms)(milliseconds to wait=u32 100) -> ()  [unwired: 1 out]
            n273 = disable-structure shown="Enabled" {
              disable-tunnel: [w360 w361] -> w350
              frame Enabled {
                n274 = property on="editSpeed" class="DigNum (strict)"() -> ("Value"=w360:dbl)  [unwired: 2 in, 2 out]
              }
              frame Disabled {
                n275 = property on="velocidade" class="DigNum (strict)"() -> ("Value"=w361:u32)  [unwired: 2 in, 2 out]
              }
            }
            n276 = property on="editSetLowerLimit" class="DigNum (strict)"() -> ("Value"=w352:u32)  [unwired: 2 in, 2 out]
            n277 = Less Or Equal?(x=w350, y=w352) -> (x <= y?=w356:bool)
            n278 = case shown="True" w356 {
              selector: w356 -> [w362 _]
              tunnel: [w362 w363] -> w354
              frame False {
              }
              frame True {
                n279 = flat-sequence {
                  tunnel: [w369] -> w364
                  tunnel: w364 -> [w373]
                  tunnel: [w372] -> w363
                  frame #0 {
                    n280 = local read "editCountLowerLimit"() -> (w368:u8)
                    n281 = Increment(x=w368) -> (x+1=w367:u8)
                    n282 = local write "editCountLowerLimit"(w367) -> ()
                    n283 = local read "editTotalLowerLimit"() -> (w366:u8)
                    n284 = Subtract(x=w366, y=w367) -> (x-y=w365:u8)
                    n285 = property on="slideWaitLowerTime" class="Slide (strict)"("Value"=w365) -> ()  [unwired: 2 in, 2 out]
                  }
                  frame #1 {
                    n286 = local read "editCountLowerLimit"() -> (w371:u8)
                    n287 = local read "editTotalLowerLimit"() -> (w370:u8)
                    n288 = Greater Or Equal?(x=w371, y=w370) -> (x >= y?=w369:bool)
                  }
                  frame #2 {
                    n289 = case shown="True" w373 {
                      selector: w373 -> [w374 w375]
                      tunnel: [w374 w375] -> w372
                      frame False {
                      }
                      frame True {
                        # "- Desliga o freio"
                        n290 = local write "ledBrake"(FALSE ("freio")) -> ()
                      }
                    }
                  }
                }
              }
            }
            n291 = Select(t=testMachine."wait " ("testMachine"), s=w354, f=testMachine."brake acquire" ("testMachine")) -> (s? t:f=w351:T2)
          }
          frame "exit" {
          }
          frame "wait " {
            # "- Aguarda 0.5s \n- Atualiza o numero de ciclos"
            n292 = flat-sequence {
              tunnel: [w390] -> w378
              frame #0 {
                n293 = local read "editCountWaitLimit"() -> (w386:u8)
                n294 = Increment(x=w386) -> (x+1=w387:u8)
                n295 = local write "editCountWaitLimit"(w387) -> ()
                n296 = local read "editTotalWaitLimit"() -> (w389:u8)
                n297 = Subtract(x=w389, y=w387) -> (x-y=w388:u8)
                n298 = property on="slideWaitTime" class="Slide (strict)"("Value"=w388) -> ()  [unwired: 2 in, 2 out]
              }
              frame #1 {
                n299 = local read "editCountWaitLimit"() -> (w392:u8)
                n300 = local read "editTotalWaitLimit"() -> (w391:u8)
                n301 = Greater Or Equal?(x=w392, y=w391) -> (x >= y?=w390:bool)
              }
            }
            n302 = disable-structure shown="Enabled" {
              frame Enabled {
                n303 = local read "ledWaitState"() -> (w399:bool)
                n304 = Not(x=w399) -> (.not. x?=w398:bool)
                n305 = local write "ledBrakeState"(FALSE ("ledBrakeState")) -> ()
                n306 = local write "ledWaitState"(w398) -> ()
              }
              frame Disabled {
              }
            }
            n307 = Wait (ms)(milliseconds to wait=u32 100) -> ()  [unwired: 1 out]
            n308 = case shown="True" w378 {
              selector: w378 -> [w393 _]
              tunnel: [w393 w397] -> w379
              frame False {
              }
              frame True {
                n309 = local read "editSetNumberOfCycles"() -> (w395:u16)
                n310 = local read "editCurrCycleCtr"() -> (w394:u32)
                n311 = Greater Or Equal?(x=w394, y=w395) -> (x >= y?=w397:bool)
                n312 = Not(x=w397) -> (.not. x?=w396:bool)
                n313 = local write "ledEnsaio"(w396) -> ()
              }
            }
            n314 = Select(t=testMachine."motor" ("testMachine"), s=w378, f=testMachine."wait " ("testMachine")) -> (s? t:f=w380:T2)
            n315 = Select(t=testMachine."finish" ("testMachine"), s=w379, f=w380) -> (s? t:f=w384:T2)
          }
        }
        n316 = disable-structure shown="Enabled" {
          frame Disabled {
          }
          frame Enabled {
            n317 = local write "ledReadyState"(FALSE ("ledReady")) -> ()
            n318 = local write "ledRunningState"(TRUE ("ledReady")) -> ()
          }
        }
        n319 = local read "buttonStart"() -> (w264:bool)
        n320 = Select(t=mainMachine."running" ("mainMachine"), s=w264, f=mainMachine."blocked" ("mainMachine")) -> (s? t:f=w261:T1)
      }
      frame "blocked" {
        n321 = local read "buttonStart"() -> (w405:bool)
        n322 = Select(t=mainMachine."ready" ("mainMachine"), s=w405, f=mainMachine."blocked" ("mainMachine")) -> (s? t:f=w401:T1)
        n323 = local write "ledRunningState"(FALSE ("ledReady")) -> ()
        n324 = local write "ledBlockState"(TRUE ("ledReady")) -> ()
      }
      frame "finish" {
        n325 = local write "ledBlockState"(FALSE ("ledReady")) -> ()
      }
    }
    "mainMachine" <- w189
    "testMachine" <- w190
  }
  n326 = disable-structure shown="Disabled" {
    frame Disabled {
    }
    frame Enabled {
    }
  }
  "velocidade" <- "velocidade 2"
